vi "Get Version.vi"(8 "error in (no error)":errorcluster, 11 "Component Configurations in":refnum<class "Component Configurations.lvclass">) -> (0 "error out":errorcluster, 2 "version":T1, 3 "Component Configurations out":refnum<class "Component Configurations.lvclass">)   [LabVIEW 2021, in "DSF Core.lvlib" / "Component Configurations.lvclass"]
uses:
  Component Configurations.lvclass
  Typedefs/DSF Version Info.ctl
  DSF Core.lvlib
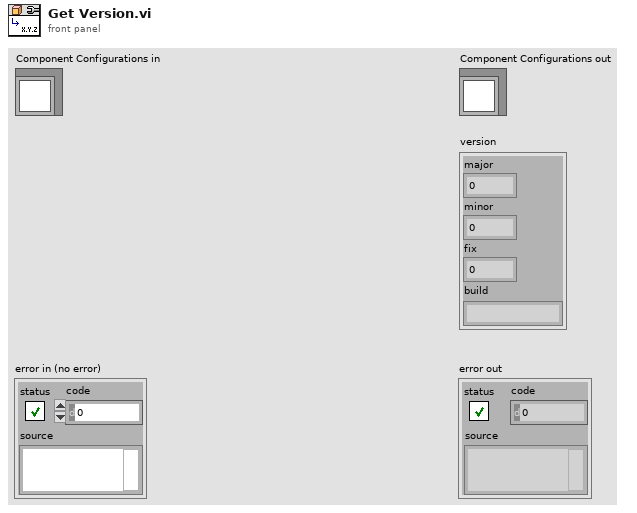
[diagram p1: front panel]
types:
  T1 = typedef "DSF Core.lvlib/DSF Version Info.ctl" = cluster{"major":u32, "minor":u32, "fix":u32, "build":string}
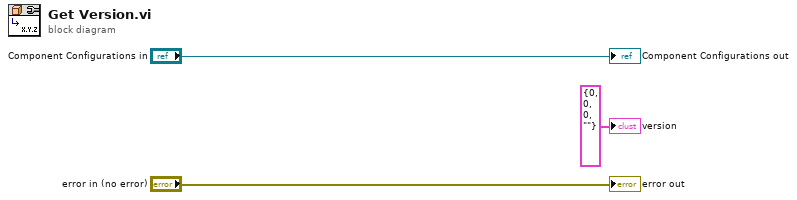
[diagram p0: block diagram]
diagram:
  "error out" <- "error in (no error)"
  "Component Configurations out" <- "Component Configurations in"
  "version" <- T1 {"major"=0, "minor"=0, "fix"=0, "build"=""} ("version")
